vi "RenameFile.vi"(8 "error in":errorcluster, 9 "replace string (\"\")":string, 10 "search string":string, 11 "appended path":path) -> (0 "error out":errorcluster)   [LabVIEW 2018]
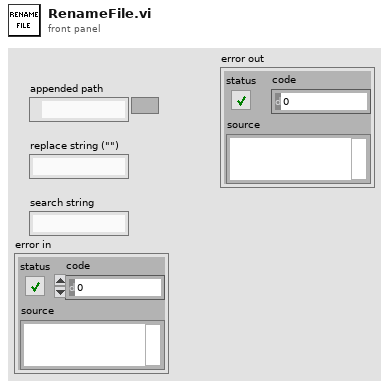
[diagram p1: front panel]
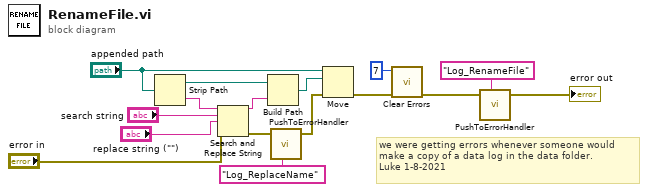
[diagram p0: block diagram]
diagram:
  # "we were getting errors whenever someone would\nmake a copy of a data log in the data folder.\nLuke 1-8-2021"
  n1 = Strip Path(path="appended path") -> (stripped path=w11:path, name=w12:string)
  n2 = Search and Replace String(input string=w12, search string="search string", replace string="replace string (\"\")", error in="error in") -> (result string=w15:string, error out=w8:errorcluster)  [unwired: 4 in, 2 out]
  n3 = Build Path(base path=w11, name or relative path=w15) -> (appended path=w16:path)
  n4 = call "PushToErrorHandler.vi"("ErrorIn"=w8, "ErrorLocation"="Log_ReplaceName") -> ("ErrorOut"=w4:errorcluster)  [unwired: 5 in]
  n5 = Move(source path="appended path", error in=w4, 10:w16) -> (error out=w7:errorcluster)  [unwired: 2 in, 2 out]
  n6 = call <vilib>:"Clear Errors.vi"("error in (no error)"=w7, "specific error code to clear (0: all)"=7) -> ("error out"=w2:errorcluster)  [unwired: 4 in, 1 out]
  n7 = call "PushToErrorHandler.vi"("ErrorIn"=w2, "ErrorLocation"="Log_RenameFile") -> ("ErrorOut"=→"error out":errorcluster)  [unwired: 5 in]
